vi "Read Data Titles.vi"(8 "error in (no error)":errorcluster, 11 "Neocera LTC-21 in":refnum<class "Neocera LTC-21.lvclass">) -> (0 "error out":errorcluster, 2 "Data titles":string[](array[string])=["Neocer_T (K)"], 3 "Neocera LTC-21 out":refnum<class "Neocera LTC-21.lvclass">)   [LabVIEW 2015, in "Neocera LTC-21.lvclass"]
uses:
  Neocera LTC-21.lvclass
  Neocera Front Panel Data.ctl
  Neocera Heater Ranges.ctl
  Neocera Set Point Aproach.ctl
  OO Devices/Device/Read Control Panel Loaded.vi
  OO Devices/Device/Read Controls Snapshot.vi
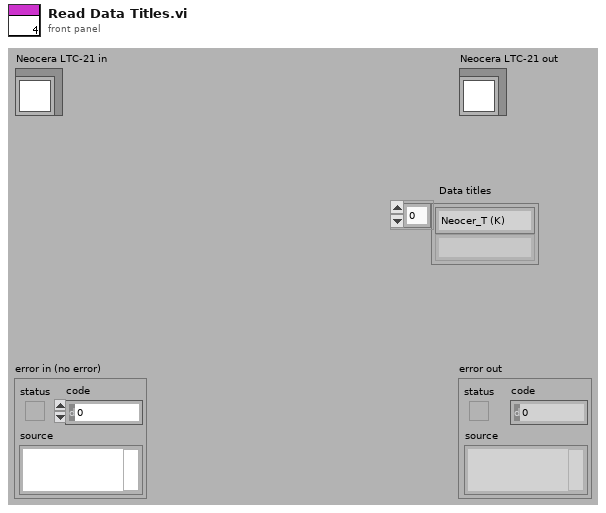
[diagram p1: front panel]
types:
  T1 = typedef "Neocera Front Panel Data.ctl" = cluster{"Channels to measure":dbl[], "Record heater":bool, "Set point":dbl, "Set Heater Range":T2, "Control":bool, "Approach":T3, "Ramp rate, K/min":dbl, "Control Channel":i16, "P":dbl, "I":dbl, "D":dbl, "Suspend heater":bool}
  T2 = typedef "Neocera Heater Ranges.ctl" = enum16{"Off", "0.05W", "0.5W", "5W", "50W"}
  T3 = typedef "Neocera Set Point Aproach.ctl" = enum16{"Instant", "Ramp"}
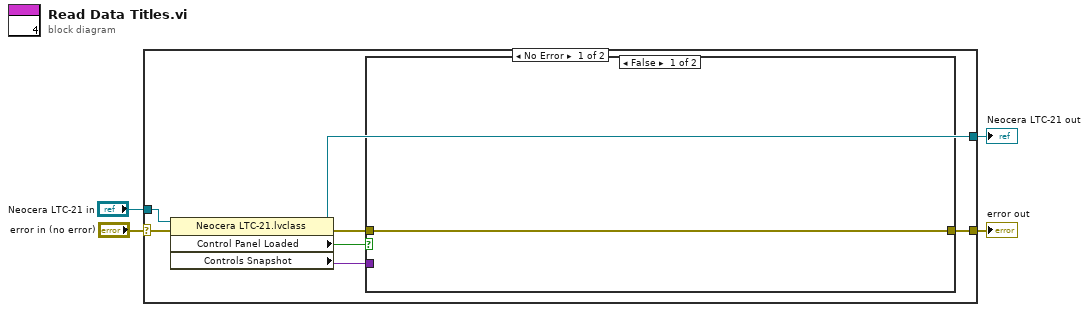
[diagram p0: block diagram]
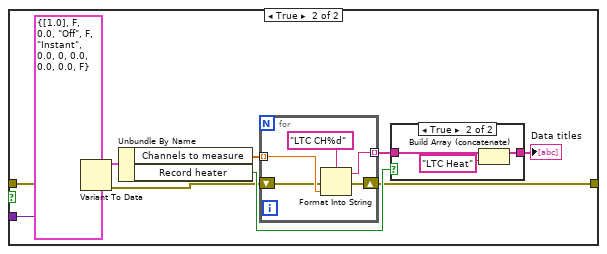
[diagram p2: hidden frame]
diagram:
  n1 = case shown="No Error" "error in (no error)" {
    selector: "error in (no error)" -> [w9 w33]
    tunnel: [w7 w33] -> w3
    tunnel: [w10 w32] -> w1
    tunnel: "Neocera LTC-21 in" -> [w11 w32]
    frame No Error {
      n2 = property class="Neocera LTC-21.lvclass"(reference=w11, error in=w9) -> (reference out=w10:refnum<class "Neocera LTC-21.lvclass">, error out=w8:errorcluster, "Control Panel Loaded"=w5:bool, "Controls Snapshot"=w6:variant)
      n3 = case shown="False" w5 {
        tunnel: w8 -> [w12 w21]
        tunnel: [w12 w14] -> w7
        tunnel: w6 -> [_ w13]
        frame False {
        }
        frame True {
          n4 = Variant To Data(error in=w21, type=T1 {"Channels to measure"=[1.0], "Record heater"=FALSE, "Set point"=0.0, "Set Heater Range"=enum."Off", "Control"=FALSE, "Approach"=enum."Instant", "Ramp rate, K/min"=0.0, "Control Channel"=0, "P"=0.0, "I"=0.0, "D"=0.0, "Suspend heater"=FALSE} ("Front Panel Data"), Variant=w13) -> (data=w20:T1, error out=w15:errorcluster)
          n5 = Unbundle By Name(w20) -> ("Channels to measure"=w19:dbl[], "Record heater"=w18:bool)
          n6 = for {
            tunnel: w19 -> [w30] mode=indexing
            tunnel: [w29] -> w17 mode=indexing
            shift-right: [w27] -> w14
            shift-left: w15 -> [w28]
            n7 = Format Into String(format string="LTC CH%d", error in=w28, w30) -> (resulting string=w29:string, error out=w27:errorcluster)  [unwired: 1 in]
          }
          n8 = case shown="True" w18 {
            tunnel: w17 -> [w23 w26]
            tunnel: [w23 w25] -> w16
            frame False {
            }
            frame True {
              n9 = Build Array (concatenate)(w26, "LTC Heat" ("format string")) -> (w25:string[])
            }
          }
          "Data titles" <- w16
        }
      }
    }
    frame Error {
    }
  }
  "error out" <- w3
  "Neocera LTC-21 out" <- w1
